vi "WM_CAP - Clipboard to LV.vi"(11 "error in (no error)":errorcluster, 13 "Erase Clipboard?":bool) -> (8 "LV_Image":T1, 15 "error out":errorcluster)   [LabVIEW 2022 SP3]
uses:
  <vilib>/picture/picture.llb/imagedata.ctl
  user32.dll
  kernel32.dll
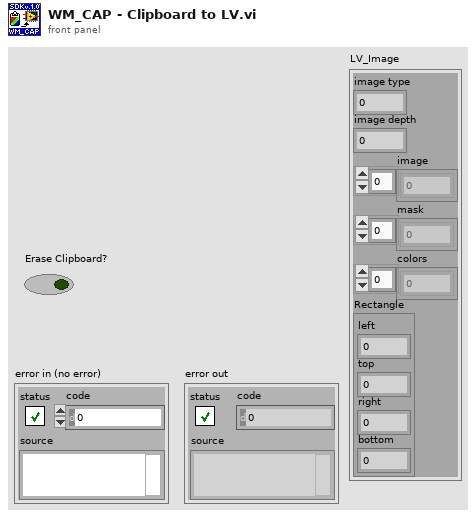
[diagram p1: front panel]
types:
  T1 = typedef "imagedata.ctl" = cluster{"image type":i32, "image depth":i32, "image":u8[], "mask":u8[], "colors":u32[], "Rectangle":cluster{"left":i16, "top":i16, "right":i16, "bottom":i16}}
  T2 = enum32{"invalid", "CF_TEXT", "CF_BITMAP", "CF_METAFILEPICT", "CF_SYLK", "CF_DIF", "CF_TIFF", "CF_OEMTEXT", "CF_DIB", "CF_PALETTE", "CF_PENDATA", "CF_RIFF", "CR_WAVE", "CF_UNICODETEXT", "CF_ENHMETAFILE", "CF_HDROP", "CF_LOCALE", "CF_DIBV5"}
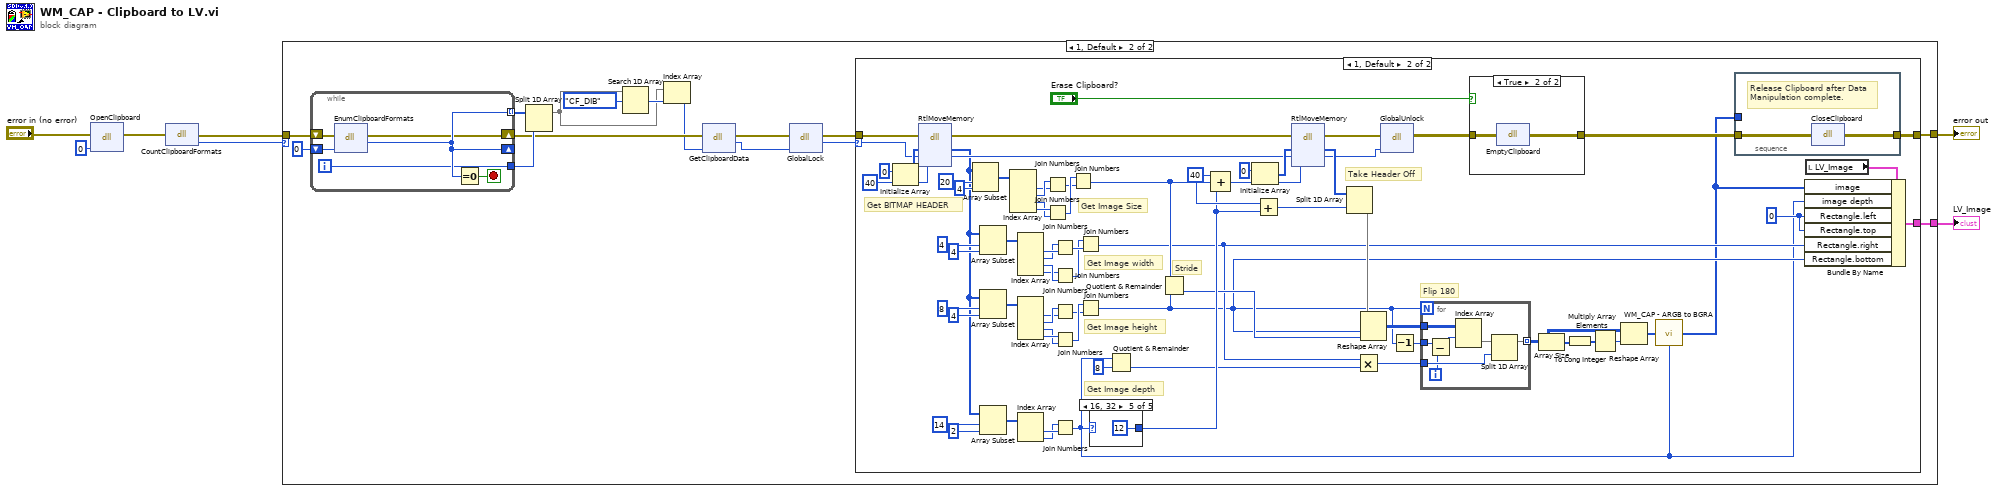
[diagram p0: block diagram]
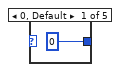
[diagram p4: hidden frame]
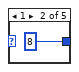
[diagram p5: hidden frame]
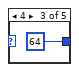
[diagram p6: hidden frame]
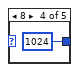
[diagram p7: hidden frame]
diagram:
  n1 = dll-call lib="user32.dll" fn="OpenClipboard"(error in="error in (no error)", "hWnd"=u32 0) -> (error out=w5:errorcluster)  [unwired: 4 in, 1 out]
  n2 = dll-call lib="user32.dll" fn="CountClipboardFormats"(error in=w5) -> (error out=w3:errorcluster, "return type"=w4:u32)  [unwired: 2 in, 1 out]
  n3 = case shown="1, Default" w4 {
    tunnel: w3 -> [w8 w22]
    tunnel: [w8 w11] -> w1
    tunnel: [_ w10] -> w2
    frame 0 {
    }
    frame 1, Default {
      n4 = while {
        shift-right: [w118] -> _
        shift-left: u32 0 -> [w120]
        shift-right: [w115] -> w18
        shift-left: w22 -> [w116]
        tunnel: [w118] -> w21 mode=indexing
        tunnel: [w117] -> w20
        i -> [w117]
        stop <- w119 stop-if-true
        n5 = dll-call lib="user32.dll" fn="EnumClipboardFormats"(error in=w116, "format"=w120) -> (error out=w115:errorcluster, "return type"=w118:u32)  [unwired: 3 in, 1 out]
        n6 = Equal To 0?(x=w118) -> (x = 0?=w119:bool)
      }
      n7 = Split 1D Array(array=w21, index=w20) -> (first subarray=w9:u32[])  [unwired: 1 out]
      n8 = Search 1D Array(1D array=w9, element=T2."CF_DIB" ("format")) -> (index of element=w17:i32)  [unwired: 1 in]
      n9 = Index Array(array=w9, index=w17) -> (element=w16:u32)
      n10 = dll-call lib="user32.dll" fn="GetClipboardData"(error in=w18, "hWnd"=w16) -> (error out=w14:errorcluster, "return type"=w15:u32)  [unwired: 3 in, 1 out]
      n11 = dll-call lib="kernel32.dll" fn="GlobalLock"(error in=w14, "hWnd"=w15) -> (error out=w12:errorcluster, "return type"=w13:u32)  [unwired: 3 in, 1 out]
      n12 = case shown="1, Default" w13 {
        selector: w13 -> [_ w93]
        tunnel: w12 -> [w24 w95]
        tunnel: [w24 w77] -> w11
        tunnel: [_ w76] -> w10
        frame 0 {
        }
        frame 1, Default {
          w44 = u32 40 ("value")
          w56 = i16 0 ("Rectangle.left")
          w94 = 40 ("dimension size")
          # "Flip 180"
          # "Stride"
          # "Get Image depth"
          # "Get Image height"
          # "Get Image width"
          # "Take Header Off"
          # "Get Image Size"
          # "Get BITMAP HEADER"
          n13 = Initialize Array(u8 0 ("element"), w94) -> (w97:u8[])
          n14 = dll-call lib="kernel32.dll" fn="RtlMoveMemory"(error in=w95, "source"=w97, "dest"=w93, "size"=w94) -> (error out=w86:errorcluster, "source"=w50:u8[], "dest"=w83:u32)  [unwired: 4 in, 1 out]
          n15 = Array Subset(array=w50, index=20, length=4) -> (w80:u8[])
          n16 = Array Subset(array=w50, index=4, length=4) -> (w74:u8[])
          n17 = Array Subset(array=w50, index=8, length=4) -> (w57:u8[])
          n18 = Array Subset(array=w50, index=14, length=2) -> (w55:u8[])
          n19 = Index Array(array=w80) -> (element #1=w89:u8, element #2=w90:u8, element #3=w91:u8, element #4=w92:u8)  [unwired: 4 in]
          n20 = Index Array(array=w74) -> (element #1=w69:u8, element #2=w68:u8, element #3=w67:u8, element #4=w66:u8)  [unwired: 4 in]
          n21 = Index Array(array=w57) -> (element #1=w62:u8, element #2=w63:u8, element #3=w64:u8, element #4=w65:u8)  [unwired: 4 in]
          n22 = Index Array(array=w55) -> (element #1=w52:u8, element #2=w51:u8)  [unwired: 2 in]
          n23 = Join Numbers(hi=w90, lo=w89) -> ((hi.lo)=w87:u16)
          n24 = Join Numbers(hi=w92, lo=w91) -> ((hi.lo)=w88:u16)
          n25 = Join Numbers(hi=w68, lo=w69) -> ((hi.lo)=w71:u16)
          n26 = Join Numbers(hi=w66, lo=w67) -> ((hi.lo)=w70:u16)
          n27 = Join Numbers(hi=w63, lo=w62) -> ((hi.lo)=w60:u16)
          n28 = Join Numbers(hi=w65, lo=w64) -> ((hi.lo)=w61:u16)
          n29 = Join Numbers(hi=w51, lo=w52) -> ((hi.lo)=w25:u16)
          n30 = Join Numbers(hi=w88, lo=w87) -> ((hi.lo)=w37:u32)
          n31 = Join Numbers(hi=w70, lo=w71) -> ((hi.lo)=w31:u32)
          n32 = Join Numbers(hi=w61, lo=w60) -> ((hi.lo)=w29:u32)
          n33 = case shown="16, 32" w25 {
            tunnel: [0 ("32bit integer") 8 ("32bit integer") 64 ("32bit integer") 1024 ("32bit integer") 12 ("32bit integer")] -> w43
            frame 0, Default {
            }
            frame 1 {
            }
            frame 4 {
            }
            frame 8 {
            }
            frame 16, 32 {
            }
          }
          n34 = Quotient & Remainder(x=w25, y=u16 8) -> (floor(x/y)=w32:u16)  [unwired: 1 out]
          n35 = Quotient & Remainder(x=w37, y=w29) -> (floor(x/y)=w35:u32)  [unwired: 1 out]
          n36 = Compound Arithmetic op=ADD(w44, w37, w43) -> (w45:u32)
          n37 = Initialize Array(u8 0 ("element"), w45) -> (w84:u8[])
          n38 = Add(x=w44, y=w43) -> (x+y=w42:u32)
          n39 = dll-call lib="kernel32.dll" fn="RtlMoveMemory"(error in=w86, "source"=w84, "dest"=w83, "size"=w45) -> (error out=w79:errorcluster, "source"=w75:u8[], "dest"=w46:u32)  [unwired: 4 in, 1 out]
          n40 = Split 1D Array(array=w75, index=w42) -> (second subarray=w36:u8[])  [unwired: 1 out]
          n41 = Multiply(x=w31, y=w32) -> (x*y=w30:u32)
          n42 = Reshape Array(w36, w29, w35) -> (w34:u8[][])
          n43 = dll-call lib="kernel32.dll" fn="GlobalUnlock"(error in=w79, "handle"=w46) -> (error out=w49:errorcluster)  [unwired: 4 in, 1 out]
          n44 = Decrement(x=w29) -> (x-1=w28:u32)
          n45 = for {
            N: w29 -> [_]
            tunnel: w34 -> [w102]
            tunnel: [w104] -> w33 mode=indexing
            tunnel: w30 -> [w103]
            tunnel: w28 -> [w100]
            i -> [w99]
            n46 = Subtract(x=w100, y=w99) -> (x-y=w98:u32)
            n47 = Index Array(array=w102, index (row)=w98) -> (element=w101:u8[])  [unwired: 1 in]
            n48 = Split 1D Array(array=w101, index=w103) -> (first subarray=w104:u8[])  [unwired: 1 out]
          }
          n49 = case shown="True" "Erase Clipboard?" {
            tunnel: w49 -> [w112 w114]
            tunnel: [w112 w113] -> w48
            frame False {
            }
            frame True {
              n50 = dll-call lib="user32.dll" fn="EmptyClipboard"(error in=w114) -> (error out=w113:errorcluster)  [unwired: 3 in, 1 out]
            }
          }
          n51 = Array Size(array=w33) -> (size(s)=w38:i32[])
          n52 = To Long Integer(number=w38) -> (32bit integer=w39:i32[])
          n53 = Multiply Array Elements(1:w39) -> (0:w40:i32)
          n54 = Reshape Array(w33, w40) -> (w27:u8[])
          n55 = call "WM_CAP - ARGB to BGRA.vi"("ARGB"=w27, "Image Depth"=w25) -> ("BGRA"=w26:u8[])  [unwired: 13 in]
          n56 = stacked-sequence {
            tunnel: [w111] -> w77
            tunnel: w48 -> [w110]
            tunnel: w26 -> [_]
            frame #0 {
              # "Release Clipboard after Data\nManipulation complete."
              n57 = dll-call lib="user32.dll" fn="CloseClipboard"(error in=w110) -> (error out=w111:errorcluster)  [unwired: 3 in, 1 out]
            }
          }
          n58 = local read "LV_Image"() -> (w78:T1)
          n59 = Bundle By Name(cluster=w78, "image"=w26, "image depth"=w25, "Rectangle.left"=w56, "Rectangle.top"=w56, "Rectangle.right"=w31, "Rectangle.bottom"=w29) -> (w76:T1)
        }
      }
    }
  }
  "LV_Image" <- w2
  "error out" <- w1
